vi "Écrire UI.vi"(10 "Framework d'acteur:Objet ajoutant des msgs à la file":refnum<class "Message Enqueuer.lvclass">, 11 "Cooler en entrée":refnum<class "Cooler.lvclass">) -> (3 "Cooler en sortie":refnum<class "Cooler.lvclass">)   [LabVIEW 2015, in "Cooler.lvlib" / "Cooler.lvclass"]
uses:
  Cooler.lvclass
  <vilib>/ActorFramework/Message Enqueuer/Message Enqueuer.lvclass
  Cooler.lvclass/Cooler.ctl
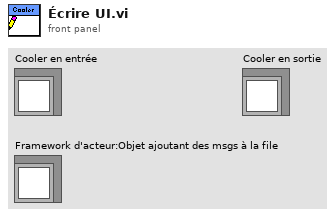
[diagram p1: front panel]
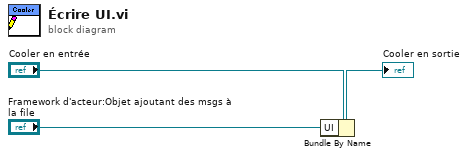
[diagram p0: block diagram]
diagram:
  n1 = Bundle By Name(cluster="Cooler en entrée", "UI"="Framework d'acteur:Objet ajoutant des msgs à la file") -> (→"Cooler en sortie":refnum<class "Cooler.lvclass">)
